vi "RSZVB Set Type Of Advanced Power Transfer Model.vi"(8 "error in (no error)":errorcluster {"code" format="%.0x"}, 9 "Model Type (Linear Approximation)":i32(ring)=1 items=["Data Set", "Linear Approximation", "Electronic Attenuator Only", "None or Mechanical Attenuator"], 10 "Channel (1)":i32=1, 11 "VISA session":refnum<visa-resource-name>) -> (0 "error out":errorcluster {"code" format="%.0x"}, 3 "dup VISA session":refnum<visa-resource-name>)   [LabVIEW 2011]
doc: "This VI selects the type of advanced power transfer model.\n\nNote(s):This VI overwrites the port specific setting; see\nSOURce<Ch>:POWer<Pt>:CONVerter:TRANsfer:DESCription.\n\nRemote-control command(s):\n[SENSe<Ch>:]CONVerter:DESCription NONE | ELECtronic | DSET | LAPProx"
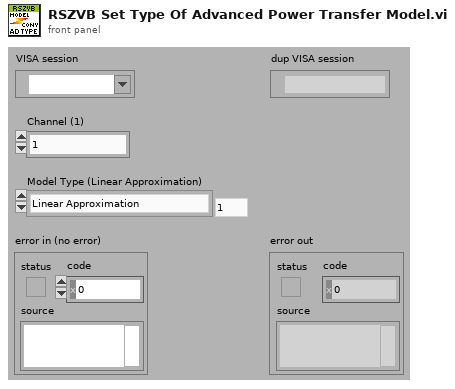
[diagram p1: front panel]
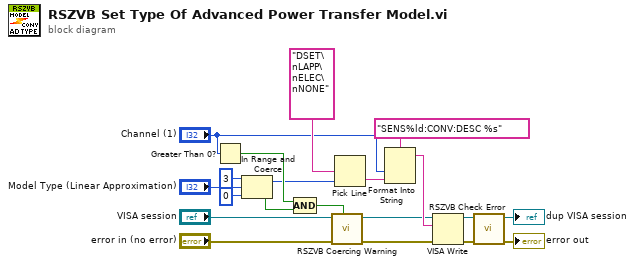
[diagram p0: block diagram]
diagram:
  n1 = Greater Than 0?(x="Channel (1)") -> (x > 0?=w16:bool)
  n2 = In Range and Coerce(upper limit=3, x="Model Type (Linear Approximation)", lower limit=0) -> (coerced(x)=w9:i32, In Range?=w15:bool)
  n3 = Compound Arithmetic op=AND(w16, w15) -> (w17:bool)
  n4 = call "RSZVB Coercing Warning.vi"("In Range?"=w17, "error in (no error)"="error in (no error)", "VISA session"="VISA session") -> ("error out"=w11:errorcluster, "dup VISA session"=w10:refnum<visa-resource-name>)  [unwired: 7 in]
  n5 = Pick Line(multi-line string="DSET\nLAPP\nELEC\nNONE", line index=w9) -> (output string=w14:string)  [unwired: 1 in]
  n6 = Format Into String(format string="SENS%ld:CONV:DESC %s", "Channel (1)", w14) -> (resulting string=w18:string)  [unwired: 2 in, 1 out]
  n7 = VISA Write(VISA resource name=w10, write buffer=w18, error in (no error)=w11) -> (VISA resource name out=w13:refnum<visa-resource-name>, error out=w12:errorcluster)  [unwired: 1 out]
  n8 = call "RSZVB Check Error.vi"("error in (no error)"=w12, "VISA session"=w13) -> ("error out"=→"error out":errorcluster, "dup VISA session"=→"dup VISA session":refnum<visa-resource-name>)  [unwired: 8 in]
